vi "SaveControlValues.vi"(6 "error in":errorcluster, 9 "path (VI name)":path) -> (0 "error out":errorcluster)   [LabVIEW 2009]
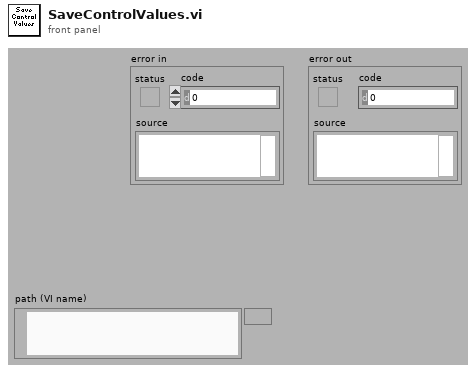
[diagram p1: front panel]
types:
  T1 = cluster{"Name":string, "type string":i16[], "data string":string}
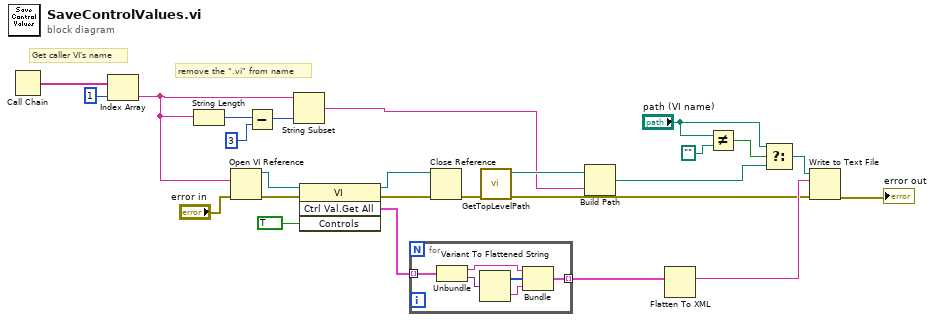
[diagram p0: block diagram]
diagram:
  # "Get caller VI's name"
  # "remove the \".vi\" from name"
  n1 = Call Chain() -> (call chain=w11:string[])
  n2 = Index Array(array=w11, index=1) -> (element=w9:string)
  n3 = String Length(string=w9) -> (length=w20:i32)
  n4 = Open VI Reference(vi path=w9, error in (no error)="error in") -> (vi reference=w8:refnum<vi>, error out=w4:errorcluster)  [unwired: 4 in]
  n5 = Subtract(x=w20, y=3) -> (x-y=w18:i32)
  n6 = String Subset(string=w9, length (rest)=w18) -> (substring=w1:string)  [unwired: 1 in]
  n7 = invoke class="VI" method="Ctrl Val.Get All"(reference=w8, error in=w4, "Controls"=TRUE ("Save control values")) -> (reference out=w7:refnum<vi>, error out=w6:errorcluster, "Get All Control Values Variant"=w23:cluster{"Name":string, "Variant Data":variant}[])  [unwired: 1 in, 1 out]
  n8 = for {
    tunnel: w23 -> [w31] mode=indexing
    tunnel: [w29] -> w22 mode=indexing
    n9 = Unbundle(w31) -> ("Name"=w30:string, "Variant Data"=w28:variant)
    n10 = Variant To Flattened String(Variant=w28) -> (data string=w26:string, 1:w27:i16[])
    n11 = Bundle("Name"=w30, "type string"=w27, "data string"=w26) -> (w29:T1)  [unwired: 1 out]
  }
  n12 = Close Reference(reference=w7, error in (no error)=w6) -> (error out=w3:errorcluster)
  n13 = call "GetTopLevelPath.vi"("error in"=w3) -> ("error out"=w2:errorcluster, "path"=w5:path)  [unwired: 9 in]
  n14 = Build Path(base path=w5, name or relative path=w1) -> (appended path=w14:path)
  n15 = Flatten To XML(anything=w22) -> (xml string=w24:string)
  n16 = Not Equal?(x="path (VI name)", y=path "") -> (x != y?=w17:bool)
  n17 = Select(t="path (VI name)", s=w17, f=w14) -> (s? t:f=w13:path)
  n18 = Write to Text File(file (use dialog)=w13, text=w24, error in=w2) -> (error out=→"error out":errorcluster)  [unwired: 3 out]
